vi "путь для общего отчета.vi"() -> (3 "path_out 2":string)   [LabVIEW 2016, in "Library.lvlib"]
uses:
  Granule-2000AT/PC/Library.lvlib
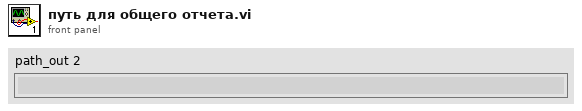
[diagram p1: front panel]
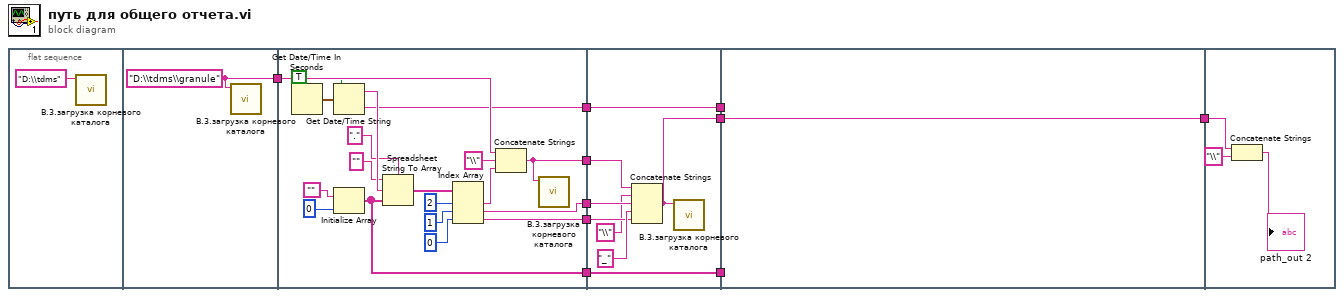
[diagram p0: block diagram]
diagram:
  n1 = flat-sequence {
    tunnel: [w12] -> w10
    tunnel: w10 -> [w23]
    tunnel: [w18] -> w9
    tunnel: [w17] -> w8
    tunnel: [w16] -> w7
    tunnel: [w15] -> w6
    tunnel: [w14] -> w5
    tunnel: w9 -> [w39]
    tunnel: w8 -> [w37]
    tunnel: w7 -> [w35]
    tunnel: [w34] -> w4
    tunnel: w6 -> [w34]
    tunnel: [w33] -> w3
    tunnel: w5 -> [w33]
    tunnel: [w32] -> w2
    tunnel: w4 -> [_]
    tunnel: w3 -> [_]
    tunnel: w2 -> [w40]
    tunnel: [w40] -> w1
    tunnel: w1 -> [w41]
    frame #0 {
      n2 = call "B.3.загрузка корневого каталога.vi"("path"="D:\\tdms") -> ()  [unwired: 10 in, 1 out]
    }
    frame #1 {
      w12 = "D:\\tdms\\granule" ("path")
      n3 = call "B.3.загрузка корневого каталога.vi"("path"=w12) -> ()  [unwired: 10 in, 1 out]
    }
    frame #2 {
      n4 = Get Date/Time In Seconds() -> (seconds since 1Jan1904=w31:timestamp)
      n5 = Get Date/Time String(seconds (now)=w31, want seconds? (F)=TRUE) -> (date string=w30:string, time string=w15:string)  [unwired: 1 in]
      n6 = Initialize Array("", 0 ("dimension size")) -> (w14:string[])
      n7 = Spreadsheet String To Array(delimiter (Tab)=".", format string="", spreadsheet string=w30, array type (2D Dbl)=w14) -> (array=w27:string[])
      n8 = Index Array(array=w27, index #1=2 ("index"), index #2=1 ("index"), index #3=0 ("index")) -> (element #1=w21:string, element #2=w18:string, element #3=w17:string)
      n9 = Concatenate Strings(w23, "\\" ("string"), w21) -> (w16:string)
      n10 = call "B.3.загрузка корневого каталога.vi"("path"=w16) -> ()  [unwired: 10 in, 1 out]
    }
    frame #3 {
      n11 = Concatenate Strings(w35, "\\" ("string"), w39, "_" ("string"), w37) -> (w32:string)
      n12 = call "B.3.загрузка корневого каталога.vi"("path"=w32) -> ()  [unwired: 10 in, 1 out]
    }
    frame #4 {
    }
    frame #5 {
      n13 = Concatenate Strings(w41, "\\" ("string")) -> (→"path_out 2":string)
    }
  }
